vi "HEWH_Ultramat_23.vi"(8 "error in":errorcluster, 11 "Message Queues out":T1) -> (0 "error out":errorcluster)   [LabVIEW 2023]
uses:
  Tenney/support/Message Queue/All Message Queues.ctl
  Tenney/support/Message Queue/Message Cluster.ctl
  Drivers/Omega FMA-1600A Series Gas Flow Meter/Type Definitions/FMA1600A Gas Type.ctl
  FVIR and LDO/support/Message Queue/Enqueue Message (Single).vi
  FVIR and LDO/support/Message Queue/Message Queue.lvlib
  Tenney/support/Message Queue/Tenney Message Queue.lvlib
panel:
  out "Debug":string[](array[string])
  in  "Debug":bool
  out "Loop Count":i32
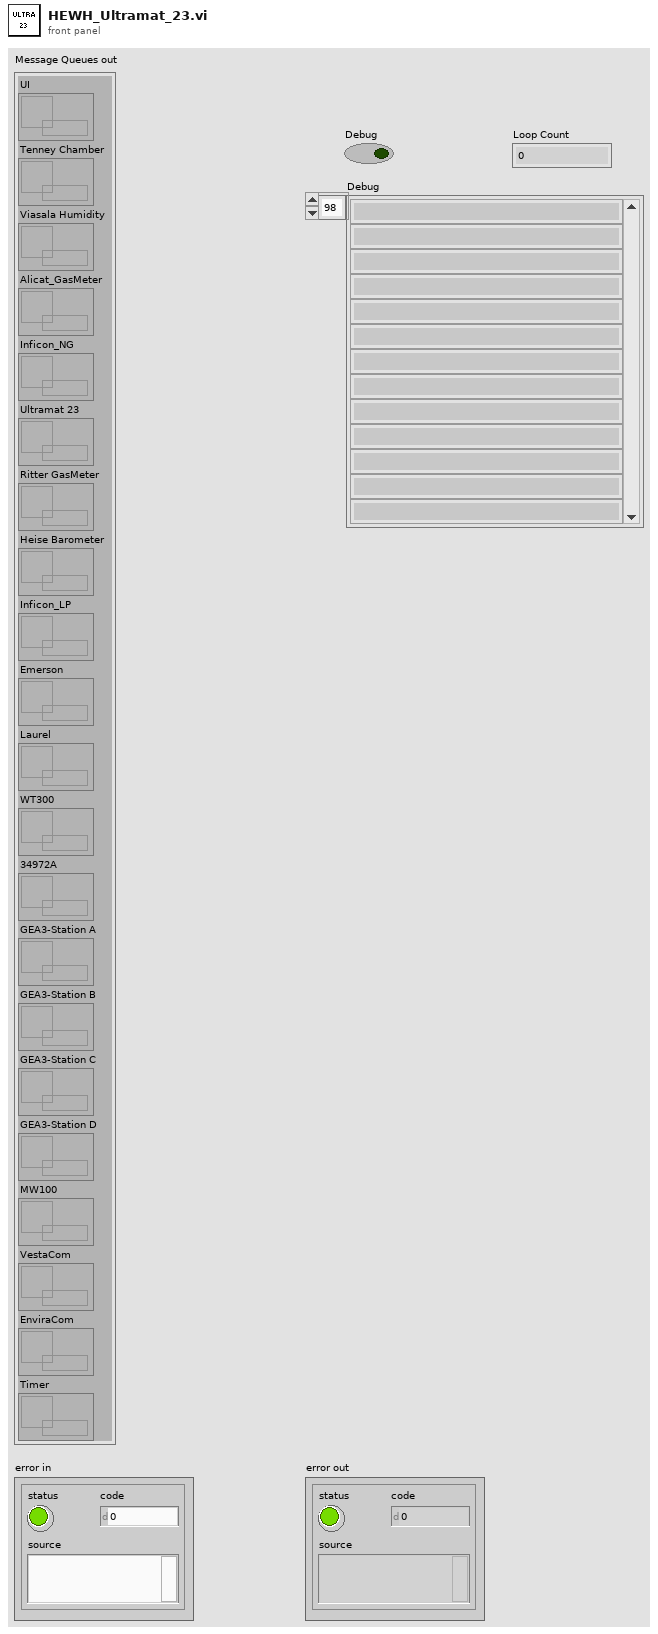
[diagram p1: front panel]
types:
  T1 = typedef "Tenney Message Queue.lvlib/All Message Queues.ctl" = cluster{"UI":refnum<queue>, "Tenney Chamber":refnum<queue>, "Viasala Humidity":refnum<queue>, "Alicat_GasMeter":refnum<queue>, "Inficon_NG":refnum<queue>, "Ultramat 23":refnum<queue>, "Ritter GasMeter":refnum<queue>, "Heise Barometer":refnum<queue>, "Inficon_LP":refnum<queue>, "Emerson":refnum<queue>, "Laurel":refnum<queue>, "WT300":refnum<queue>, "34972A":refnum<queue>, "GEA3-Station A":refnum<queue>, "GEA3-Station B":refnum<queue>, "GEA3-Station C":refnum<queue>, "GEA3-Station D":refnum<queue>, "MW100":refnum<queue>, "VestaCom":refnum<queue>, "EnviraCom":refnum<queue>, "Timer":refnum<queue>}
  T2 = typedef "FMA1600A Gas Type.ctl" = string
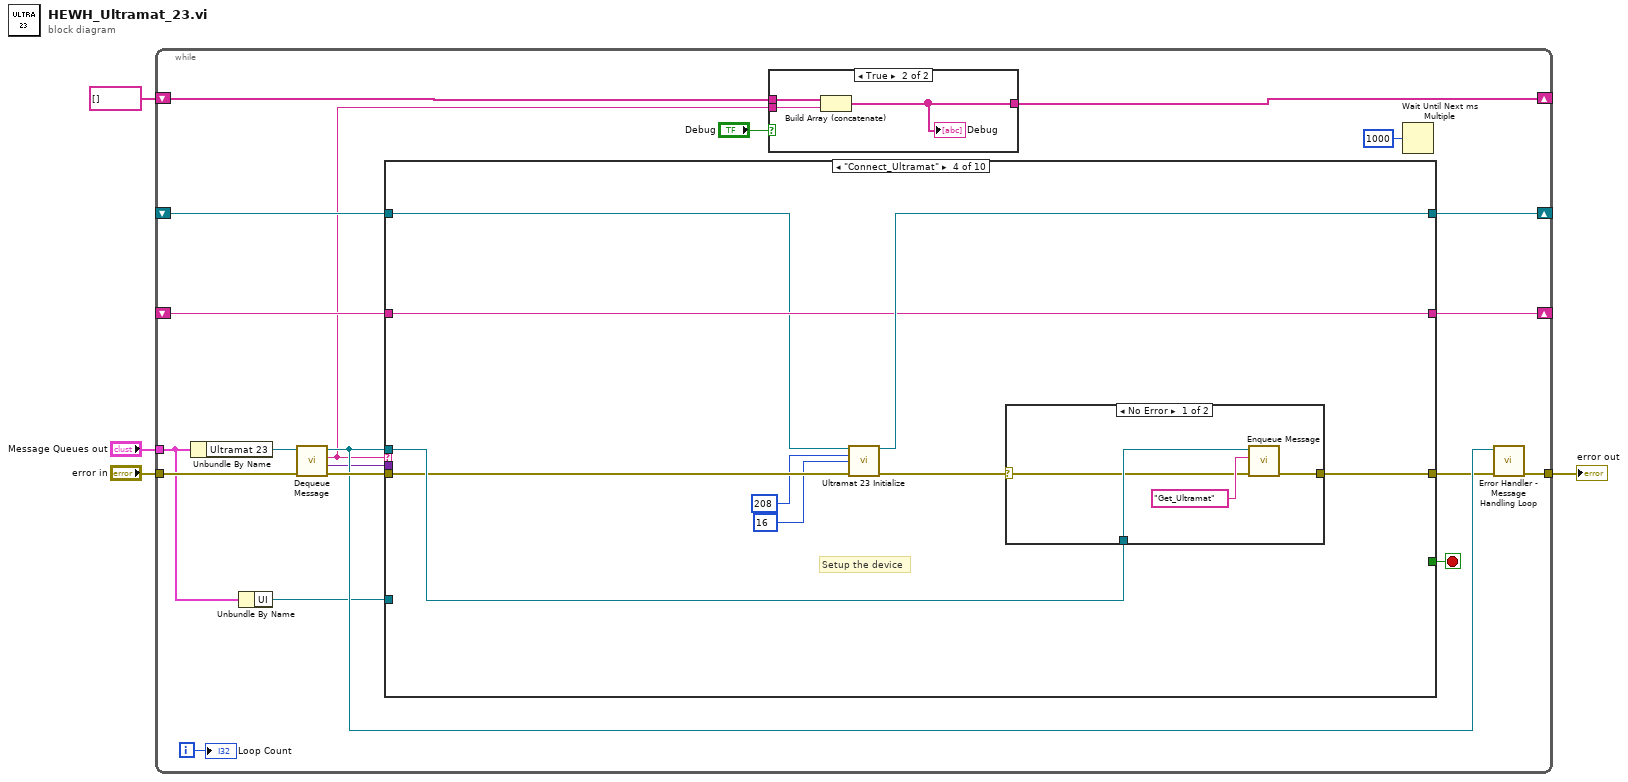
[diagram p0: block diagram]
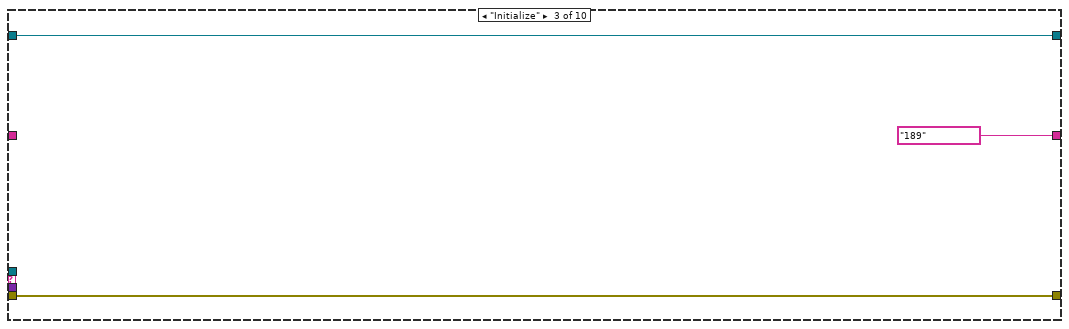
[diagram p5: hidden frame]
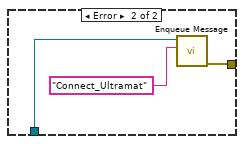
[diagram p6: hidden frame]
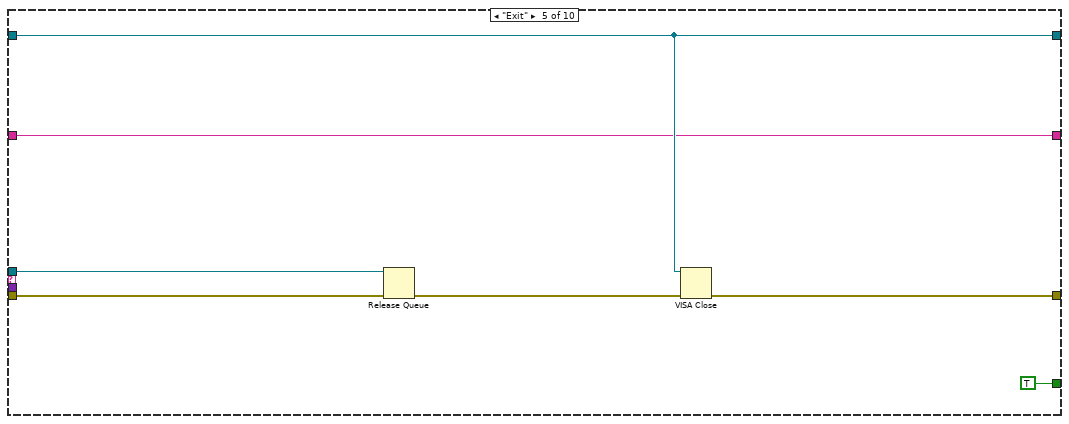
[diagram p7: hidden frame]
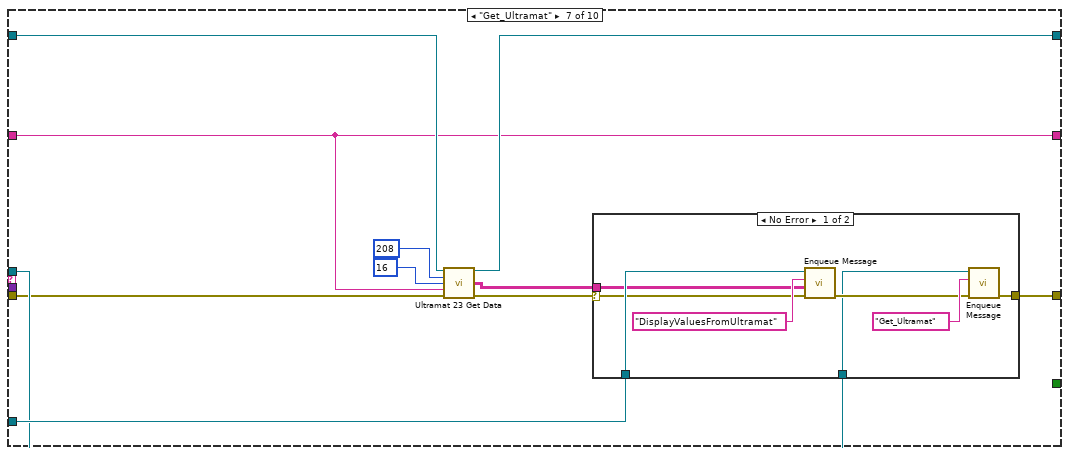
[diagram p9: hidden frame]
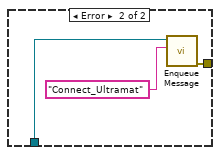
[diagram p10: hidden frame]
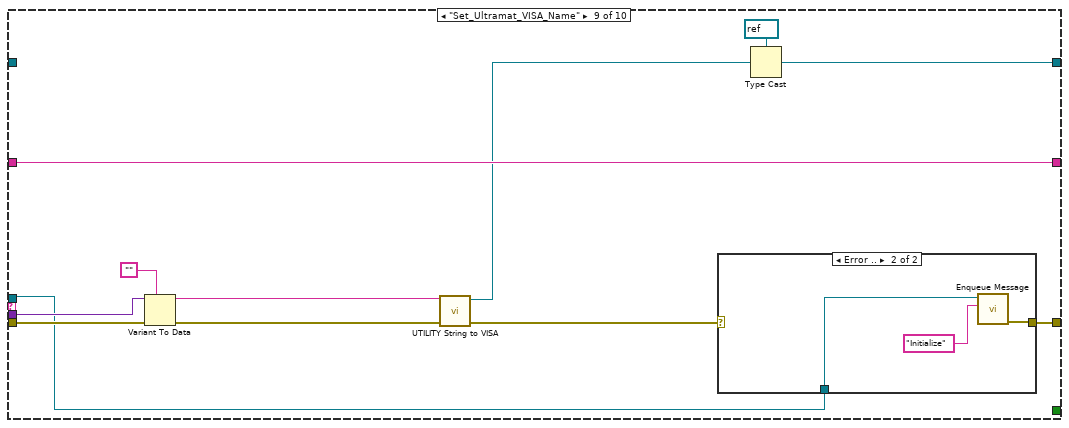
[diagram p12: hidden frame]
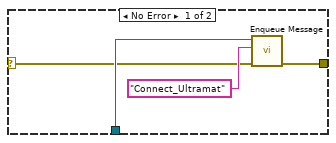
[diagram p13: hidden frame]
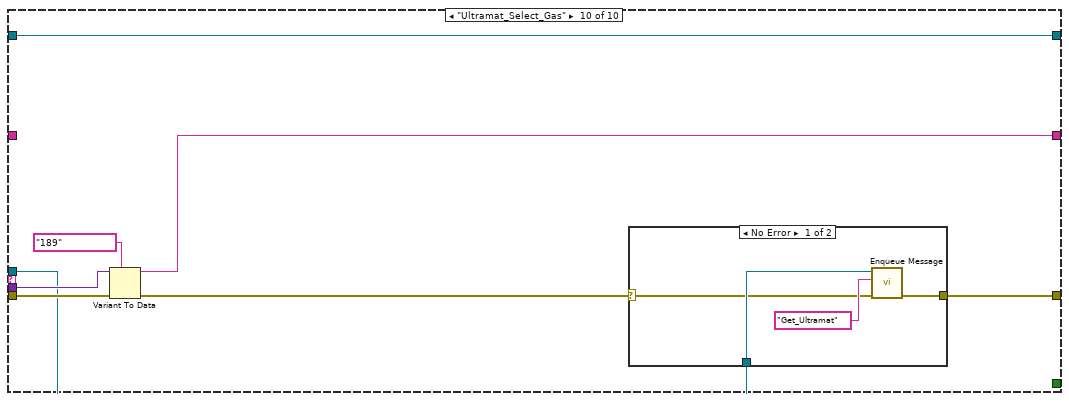
[diagram p14: hidden frame]
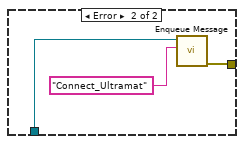
[diagram p15: hidden frame]
diagram:
  n1 = while {
    tunnel: "Message Queues out" -> [w16]
    tunnel: "error in" -> [w23]
    tunnel: [w19] -> w3
    shift-right: [w14] -> _
    shift-left: _ -> [w13]
    shift-right: [w11] -> _
    shift-left: _ -> [w10]
    shift-right: [w6] -> _
    shift-left: string[] [] -> [w7]
    i -> [w12]
    stop <- w21 stop-if-true
    n2 = Unbundle By Name(w16) -> ("Ultramat 23"=w24:refnum<queue>)
    n3 = Unbundle By Name(w16) -> ("UI"=w15:refnum<queue>)
    n4 = call "Dequeue Message.vi"("error in (no error)"=w23, "Message Queue"=w24) -> ("error out"=w22:errorcluster, "Message Data"=w9:variant, "Message"=w5:string, "dup Message Queue"=w20:refnum<queue>)  [unwired: 6 in]
    n5 = case shown="\"Connect_Ultramat\"" w5 {
      tunnel: w22 -> [w30 w33 w36 w44 w54 w62 w68 w87 w100 w114]
      tunnel: [w30 w33 w36 w46 w57 w62 w73 w87 w98 w110] -> w18
      tunnel: [_ _ _ _ TRUE _ _ _ _ _] -> w21
      tunnel: w20 -> [_ _ _ w45 w59 _ w72 _ w97 w108]
      tunnel: w15 -> [_ _ _ _ _ _ w74 _ _ _]
      tunnel: [w31 w34 w37 w43 w56 w63 w70 w88 w89 w115] -> w14
      tunnel: w13 -> [w31 w34 w37 w38 w56 w63 w71 w88 _ w115]
      tunnel: [w29 w32 T2 "189" ("Gas Type") w41 w55 w61 w64 w86 w96 w111] -> w11
      tunnel: w10 -> [w29 w32 _ w41 w55 w61 w64 w86 w96 _]
      tunnel: w9 -> [_ _ _ _ _ _ _ _ w99 w113]
      frame "---------- Setup ----------" {
      }
      frame Default {
      }
      frame "Initialize" {
      }
      frame "Connect_Ultramat" {
        # "Setup the device"
        n6 = call "Ultramat 23 Initialize.vi"("VISA resource name"=w38, "Source Address"=u8 208, "Target Address"=u8 16, "error in (no error)"=w44) -> ("VISA Session Out"=w43:refnum<visa-resource-name>, "error out"=w42:errorcluster)  [unwired: 6 in, 4 out]
        n7 = case shown="No Error" w42 {
          selector: w42 -> [w47 _]
          tunnel: [w49 w52] -> w46
          tunnel: w45 -> [w48 w51]
          frame No Error {
            n8 = call-poly "Enqueue Message.vi"("error in (no error)"=w47, "Message"="Get_Ultramat", "Message Queue"=w48) -> ("error out"=w49:errorcluster)  [unwired: 7 in, 1 out]
          }
          frame Error {
            n9 = call-poly "Enqueue Message.vi"("Message"="Connect_Ultramat", "Message Queue"=w51) -> ("error out"=w52:errorcluster)  [unwired: 8 in, 1 out]
          }
        }
      }
      frame "Exit" {
        n10 = Release Queue(queue=w59, error in (no error)=w54) -> (error out=w58:errorcluster)  [unwired: 1 in, 2 out]
        n11 = VISA Close(VISA resource name=w56, error in (no error)=w58) -> (error out=w57:errorcluster)
      }
      frame "---------- Data Collection ----------" {
      }
      frame "Get_Ultramat" {
        n12 = call "Ultramat 23 Get Data.vi"("VISA resource name"=w71, "Source Address"=u8 208, "Target Address"=u8 16, "Gas Type"=w64, "error in (no error)"=w68) -> ("VISA Session Out"=w70:refnum<visa-resource-name>, "Data Array"=w69:string[][], "error out"=w65:errorcluster)  [unwired: 6 in, 2 out]
        n13 = case shown="No Error" w65 {
          selector: w65 -> [w75 _]
          tunnel: w74 -> [w81 _]
          tunnel: [w78 w84] -> w73
          tunnel: w72 -> [w77 w83]
          tunnel: w69 -> [w76 _]
          frame No Error {
            n14 = call-poly "Enqueue Message.vi"("error in (no error)"=w75, "Message Data"=w76, "Message"="DisplayValuesFromUltramat", "Message Queue"=w81) -> ("error out"=w79:errorcluster)  [unwired: 6 in, 1 out]
            n15 = call-poly "Enqueue Message.vi"("error in (no error)"=w79, "Message"="Get_Ultramat", "Message Queue"=w77) -> ("error out"=w78:errorcluster)  [unwired: 7 in, 1 out]
          }
          frame Error {
            n16 = call-poly "Enqueue Message.vi"("Message"="Connect_Ultramat", "Message Queue"=w83) -> ("error out"=w84:errorcluster)  [unwired: 8 in, 1 out]
          }
        }
      }
      frame "---------- Events ----------" {
      }
      frame "Set_Ultramat_VISA_Name" {
        n17 = Variant To Data(error in=w100, type="", Variant=w99) -> (data=w92:string, error out=w94:errorcluster)
        n18 = call "UTILITY String to VISA.vi"("error in (no error)"=w94, "VISA Name"=w92) -> ("error out"=w93:errorcluster, "VISA resource name out"=w90:refnum<visa-resource-name>)  [unwired: 8 in]
        n19 = case shown="Error .." w93 {
          selector: w93 -> [w101 _]
          tunnel: [w103 w106] -> w98
          tunnel: w97 -> [w102 w105]
          frame No Error {
            n20 = call-poly "Enqueue Message.vi"("error in (no error)"=w101, "Message"="Connect_Ultramat", "Message Queue"=w102) -> ("error out"=w103:errorcluster)  [unwired: 7 in, 1 out]
          }
          frame Error {
            n21 = call-poly "Enqueue Message.vi"("Message"="Initialize", "Message Queue"=w105) -> ("error out"=w106:errorcluster)  [unwired: 8 in, 1 out]
          }
        }
        n22 = Type Cast(type=refnum<visa-resource-name> refnum ("VISA Session Out"), x=w90) -> (*(type *) &x=w89:refnum<visa-resource-name>)
      }
      frame "Ultramat_Select_Gas" {
        n23 = Variant To Data(error in=w114, type=T2 "189" ("Gas Type"), Variant=w113) -> (data=w111:T2, error out=w109:errorcluster)
        n24 = case shown="No Error" w109 {
          selector: w109 -> [w116 _]
          tunnel: [w118 w121] -> w110
          tunnel: w108 -> [w117 w120]
          frame No Error {
            n25 = call-poly "Enqueue Message.vi"("error in (no error)"=w116, "Message"="Get_Ultramat", "Message Queue"=w117) -> ("error out"=w118:errorcluster)  [unwired: 7 in, 1 out]
          }
          frame Error {
            n26 = call-poly "Enqueue Message.vi"("Message"="Connect_Ultramat", "Message Queue"=w120) -> ("error out"=w121:errorcluster)  [unwired: 8 in, 1 out]
          }
        }
      }
    }
    n27 = case shown="True" "Debug" {
      tunnel: w5 -> [_ w28]
      tunnel: w7 -> [w25 w27]
      tunnel: [w25 w26] -> w6
      frame False {
      }
      frame True {
        n28 = Build Array (concatenate)(w27, w28) -> (w26:string[])
        "Debug" <- w26
      }
    }
    n29 = Wait Until Next ms Multiple(millisecond multiple=u32 1000) -> ()  [unwired: 1 out]
    n30 = call "Error Handler - Message Handling Loop.vi"("error in (no error)"=w18, "Message Queue"=w20) -> ("dup error in"=w19:errorcluster)  [unwired: 8 in, 1 out]
    "Loop Count" <- w12
  }
  "error out" <- w3
